vi "MGCC_StaEst_convert_topology_p_node.vi"() -> (0 "zero_t":cdb[][][](array[numeric]))   [LabVIEW 2016]
uses:
  <vilib>/imath/engines/lvmath2/RunTimeEngine/IndexRead/NIMS M($,S).vi
  <instcachedir>/0/NIMS M($,S)_3E5749BBB62E49528D4765A77F1F6D98.lvgen/NIMS M($,S)_3E5749BBB62E49528D4765A77F1F6D98_001.vi
  <vilib>/imath/engines/lvmath2/RunTimeEngine/BuiltInFunctions/length/NIMS_length(GV).vi
  <instcachedir>/0/NIMS_length(GV)_08A3D13377FD4E4B96F5795FBF3698FA.lvgen/NIMS_length(GV)_08A3D13377FD4E4B96F5795FBF3698FA_001.vi
  <vilib>/imathl/engines/lvmath/Functions/Error Handling/Create Error.vi
  <vilib>/imath/engines/lvmath2/RunTimeEngine/RangeToken/NIMS_Range_R3 - Integer.vi
  <instcachedir>/0/NIMS_Range_R3 - Integer_A435E2FF893B4C718FD5055FE39FE2F6.lvgen/NIMS_Range_R3 - Integer_A435E2FF893B4C718FD5055FE39FE2F6_000.vi
  <vilib>/imath/engines/lvmath2/RunTimeEngine/CommandStatement/MC_CommandStatement_break.vi
  <vilib>/imath/engines/lvmath2/RunTimeEngine/IndexRead/NIMS M(S,S).vi
  <instcachedir>/0/NIMS M(S,S)_AC51E74150A542F7991B9634C66F3096.lvgen/NIMS M(S,S)_AC51E74150A542F7991B9634C66F3096_001.vi
  <vilib>/imath/engines/lvmath/Functions/Error Handling/MergeErrorsWrapper.vi
  <vilib>/imath/engines/lvmath2/RunTimeEngine/IndexRead/NIMS M(S,$).vi
  <instcachedir>/0/NIMS M(S,$)_F24F360562DE41D8BE234322A2E15C65.lvgen/NIMS M(S,$)_F24F360562DE41D8BE234322A2E15C65_001.vi
  <vilib>/imath/engines/lvmath2/RunTimeEngine/IndexReplace/NIMS M(S,$)=V.vi
  <instcachedir>/0/NIMS M(S,$)=V_BCCFA522A894489B8FA760383D74A164.lvgen/NIMS M(S,$)=V_BCCFA522A894489B8FA760383D74A164_002.vi
  <vilib>/imath/engines/lvmath2/RunTimeEngine/ErrorHandling/NIMS_Create Error From Enums.vi
  <vilib>/imath/engines/lvmath2/RunTimeEngine/NodeEndStatement/NIMS_NodeEndStatement_Output.vi
  <instcachedir>/0/NIMS_NodeEndStatement_Output_53EC0D466D134D7ABD903AC30B43404B.lvgen/NIMS_NodeEndStatement_Output_53EC0D466D134D7ABD903AC30B43404B_003.vi
  <vilib>/imath/engines/lvmath2/RunTimeEngine/ErrorHandling/NIMS_Finalize Error.vi
panel:
  out "P_node":cdb[][](array[numeric])
  out "Array":cdb[][](array[numeric])
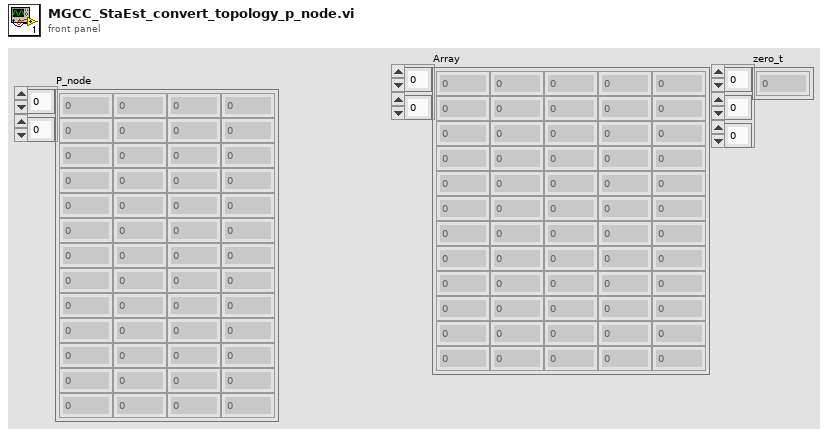
[diagram p1: front panel]
types:
  T1 = cluster{"V_node":cdb[][], "P_node":cdb[][], "I_node":cdb[][], "NumN":dbl, "NumL":dbl, "Ybus":cdb[][], "sspn":dbl[][], "ssqn":dbl[][], "ssvn":dbl[][], "SlackBus":dbl, "Topology":dbl[][]}
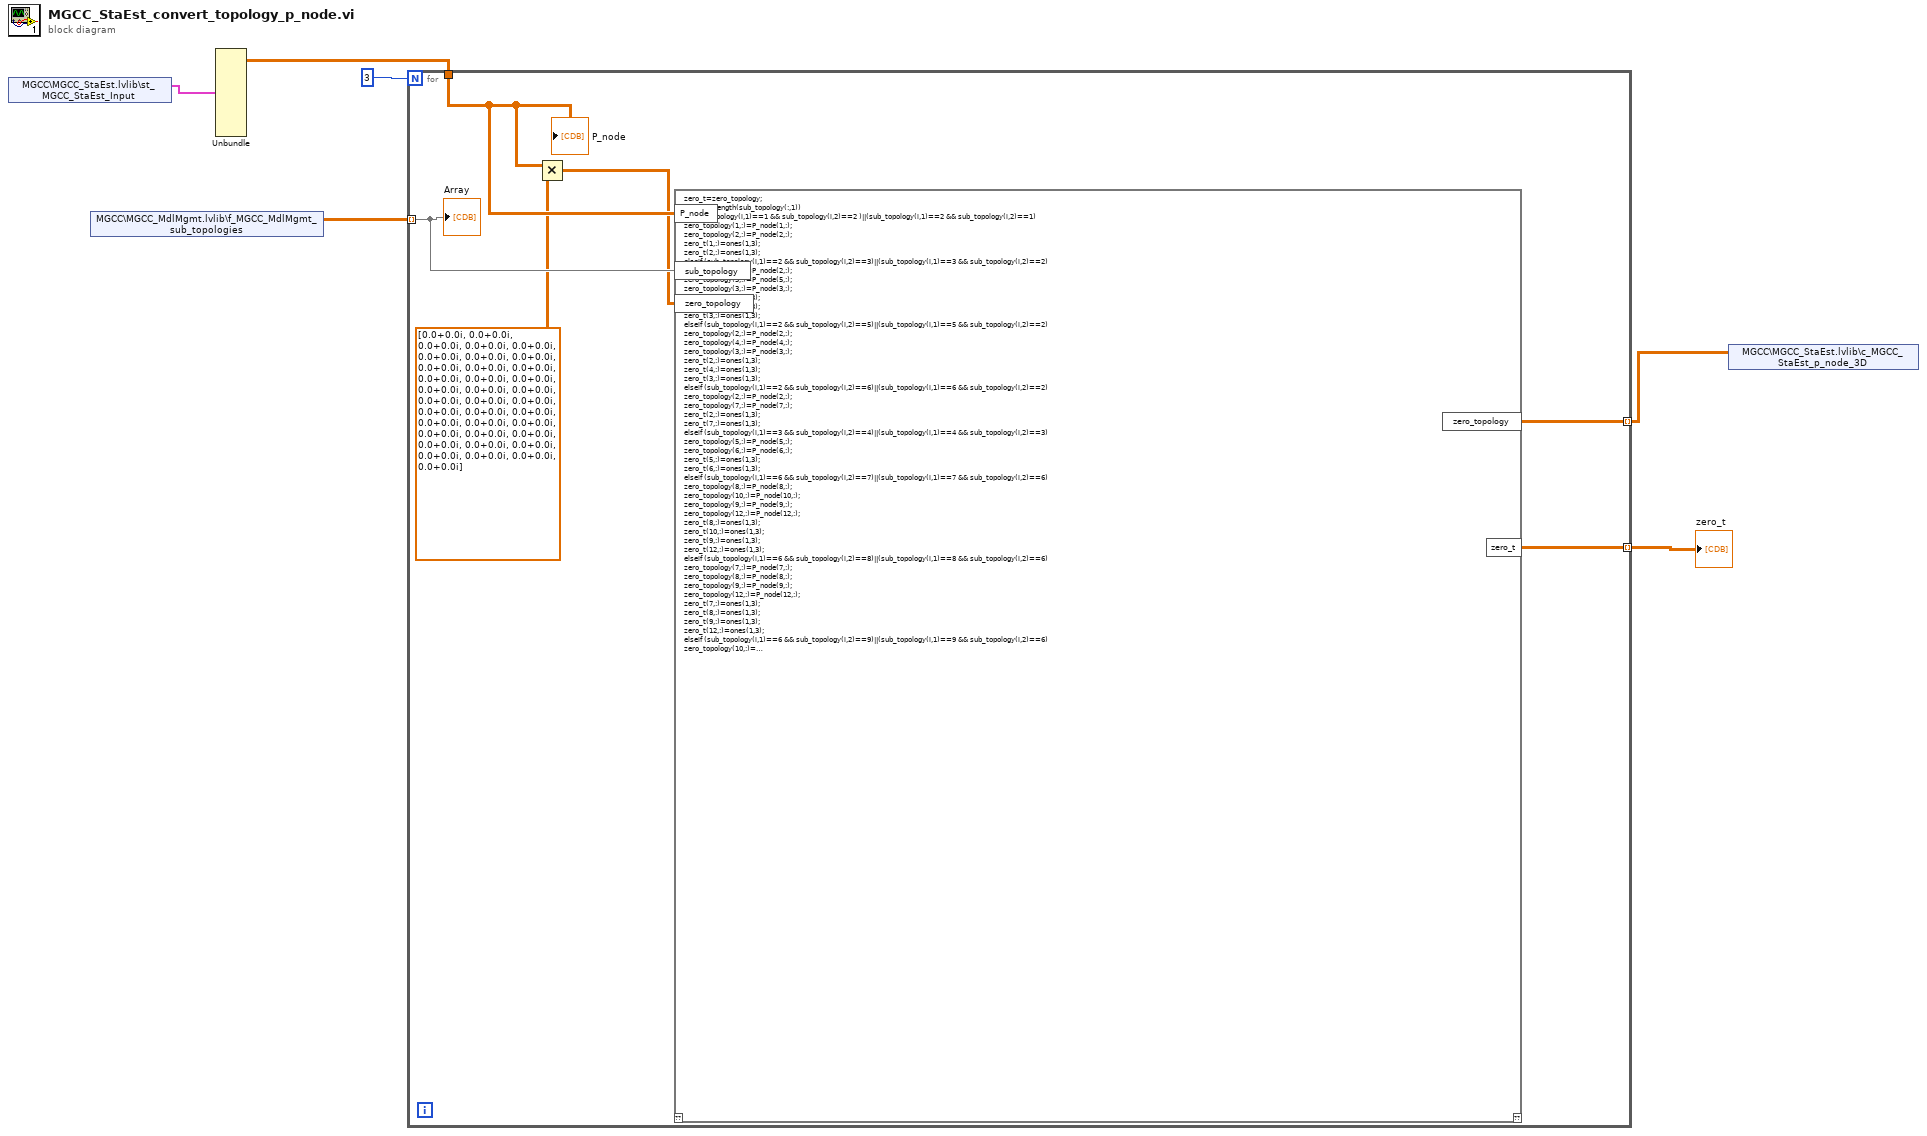
[diagram p0: block diagram]
diagram:
  n1 = shared-variable "MGCC\\MGCC_StaEst.lvlib\\st_MGCC_StaEst_Input"() -> (w4:T1)  [unwired: 1 in, 1 out]
  n2 = shared-variable "MGCC\\MGCC_MdlMgmt.lvlib\\f_MGCC_MdlMgmt_sub_topologies"() -> (w5:cdb[][][])  [unwired: 1 in, 1 out]
  n3 = Unbundle(w4) -> ("P_node"=w3:cdb[][])  [unwired: 10 out]
  n4 = for {
    N: 3 -> [_]
    tunnel: w5 -> [w12] mode=indexing
    tunnel: w3 -> [w11]
    tunnel: [w8] -> w2 mode=indexing
    tunnel: [w7] -> w1 mode=indexing
    n5 = Multiply(x=w11, y=cdb[][] [[0.0+0.0i, 0.0+0.0i, 0.0+0.0i], [0.0+0.0i, 0.0+0.0i, 0.0+0.0i], [0.0+0.0i, 0.0+0.0i, 0.0+0.0i], [0.0+0.0i, 0.0+0.0i, 0.0+0.0i], [0.0+0.0i, 0.0+0.0i, 0.0+0.0i], [0.0+0.0i, 0.0+0.0i, 0.0+0.0i], [0.0+0.0i, 0.0+0.0i, 0.0+0.0i], [0.0+0.0i, 0.0+0.0i, 0.0+0.0i], [0.0+0.0i, 0.0+0.0i, 0.0+0.0i], [0.0+0.0i, 0.0+0.0i, 0.0+0.0i], [0.0+0.0i, 0.0+0.0i, 0.0+0.0i], [0.0+0.0i, 0.0+0.0i, 0.0+0.0i]]) -> (x*y=w9:cdb[][])
    n6 = mathscript code="zero_t=zero_topology;\nfor i=1:1:length(sub_topology(:,1))\nif (sub_topology(i,1)==1 && sub_topology(i,2)==2 )||(sub_topology(i,1)==2 && sub_topology(i,2)==1)\nzero_topology(1,:)=P_node(1,:);\nzero_topology(2,:)=P_node(2,:);\nzero_t(1,:)=ones(1,3);\nzero_t(2,:)=ones(1,3);\nelseif (sub_topology(i,1)==2 && sub_topology(i,2)==3)||(sub_topology(i,1)==3 && sub_topology(i,2)==2)\nzero_topology(2,:)=P_node(2,:);\nzero_topology(5,:)=P_node(5,:);\nzero_topology(3,:)=P_node(3,:);\nzero_t(2,:)=ones(1,3);\nzero_t(5,:)=ones(1,3);\nzero_t(3,:)=ones(1,3);\nelseif (sub_topology(i,1)==2 && sub_topology(i,2)==5)||(sub_topology(i,1)==5 && sub_topology(i,2)==2)\nzero_topology(2,:)=P_node(2,:);\nzero_topology(4,:)=P_node(4,:);\nzero_topology(3,:)=P_node(3,:);\nzero_t(2,:)=ones(1,3);\nzero_t(4,:)=ones(1,3);\nzero_t(3,:)=ones(1,3);\nelseif (sub_topology(i,1)==2 && sub_topology(i,2)==6)||(sub_topology(i,1)==6 && sub_topology(i,2)==2)\nzero_topology(2,:)=P_node(2,:);\nzero_topology(7,:)=P_node(7,:);\nzero_t(2,:)=ones(1,3);\nzero_t(7,:)=ones(1,3);\nelseif (sub_topology(i,1)==3 && sub_topology(i,2)==4)||(sub_topology(i,1)==4 && sub_topology(i,2)==3)\nzero_topology(5,:)=P_node(5,:);\nzero_topology(6,:)=P_node(6,:);\nzero_t(5,:)=ones(1,3);\nzero_t(6,:)=ones(1,3);\nelseif (sub_topology(i,1)==6 && sub_topology(i,2)==7)||(sub_topology(i,1)==7 && sub_topology(i,2)==6)\nzero_topology(8,:)=P_node(8,:);\nzero_topology(10,:)=P_node(10,:);\nzero_topology(9,:)=P_node(9,:);\nzero_topology(12,:)=P_node(12,:);\nzero_t(8,:)=ones(1,3);\nzero_t(10,:)=ones(1,3);\nzero_t(9,:)=ones(1,3);\nzero_t(12,:)=ones(1,3);\nelseif (sub_topology(i,1)==6 && sub_topology(i,2)==8)||(sub_topology(i,1)==8 && sub_topology(i,2)==6)\nzero_topology(7,:)=P_node(7,:);\nzero_topology(8,:)=P_node(8,:);\nzero_topology(9,:)=P_node(9,:);\nzero_topology(12,:)=P_node(12,:);\nzero_t(7,:)=ones(1,3);\nzero_t(8,:)=ones(1,3);\nzero_t(9,:)=ones(1,3);\nzero_t(12,:)=ones(1,3);\nelseif (sub_topology(i,1)==6 && sub_topology(i,2)==9)||(sub_topology(i,1)==9 && sub_topology(i,2)==6)\nzero_topology(10,:)=P_node(10,:);\nzero_topology(11,:)=P_node(11,:);\nzero_t(10,:)=ones(1,3);\nzero_t(11,:)=ones(1,3);\nend\nend\n%if zero_t==zero_topology\n%zero_topology=zero_topology+0.01;\n%end"("P_node"=w11, "sub_topology"=w12, "zero_topology"=w9) -> ("zero_topology"=w8:cdb[][], "zero_t"=w7:cdb[][])  [unwired: 1 in, 1 out]
    "Array" <- w12
    "P_node" <- w11
  }
  "zero_t" <- w1
  n7 = shared-variable "MGCC\\MGCC_StaEst.lvlib\\c_MGCC_StaEst_p_node_3D"(w2) -> ()  [unwired: 1 in, 1 out]
